vi "Closest45rounding.vi"() -> ()   [LabVIEW 2018]
panel:
  out "NewAngle":dbl format="%#_13g"
  in  "Angle":dbl format="%#_13g"
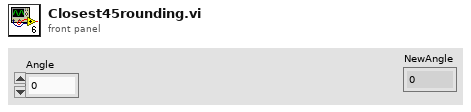
[diagram p1: front panel]
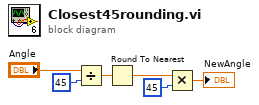
[diagram p0: block diagram]
diagram:
  n1 = Divide(x="Angle", y=45) -> (x/y=w4:dbl)
  n2 = Round To Nearest(number=w4) -> (nearest integer value=w3:dbl)
  n3 = Multiply(x=w3, y=45) -> (x*y=→"NewAngle":dbl)
